vi "MasterAquisitionFile_2P_Test.vi"() -> ()   [LabVIEW 2020]
uses:
  <vilib>/userDefined/High Color/IMAQdx.ctl
  <vilib>/vision/driver/IMAQdx.llb/IMAQdx Camera Control Mode.ctl
  <vilib>/vision/driver/IMAQdx.llb/IMAQdx Acquisition Mode.ctl
  <vilib>/vision/driver/IMAQdx.llb/IMAQdx Buffer Number Mode.ctl
  <vilib>/DAQmx/write.llb/DAQmx Write (Digital 1D Wfm NChan NSamp).vi
  <vilib>/DAQmx/read.llb/DAQmx Read (Digital 1D Bool 1Chan 1Samp).vi
  <vilib>/DAQmx/read.llb/DAQmx Read (Analog 1D Wfm NChan NSamp).vi
  <vilib>/Waveform/DWDTOps.llb/DWDT Digital to Boolean Array.vi
  <vilib>/DAQmx/create/channels.llb/DAQmx Create Channel (DO-Digital Output).vi
  <vilib>/DAQmx/configure/timing.llb/DAQmx Timing (Sample Clock).vi
  <vilib>/Waveform/DWDTOps.llb/DWDT Uncompress Digital.vi
  <vilib>/DAQmx/miscellaneous.llb/DAQmx Fill In Error Info.vi
  <vilib>/DAQmx/create/channels.llb/DAQmx Create Channel (DI-Digital Input).vi
  <vilib>/DAQmx/create/channels.llb/DAQmx Create Channel (AI-Voltage-Basic).vi
  <vilib>/DAQmx/configure/trigger.llb/DAQmx Start Trigger (Digital Edge).vi
  <vilib>/DAQmx/create/channels.llb/DAQmx Create Channel (CO-Pulse Generation-Frequency).vi
  <vilib>/DAQmx/configure/timing.llb/DAQmx Timing (Implicit).vi
  <vilib>/vision/driver/NI_Vision_Acquisition_Software.lvlib
  <resource>/objmgr/imaqdx.rc
  <resource>/objmgr/daqmx.rc
panel:
  in  "Analog Input Channels":tag="Dev2/ai0:3"
  out "Auditory":bool
  out "RPad":bool
  out "LPad":bool
  in  "Sol Stim Parameters":cluster{"Fs":dbl, "Samples":dbl}
  in  "LED Stim Parameters":cluster{"Fs":dbl, "Samples":dbl}
  in  "Generate Stimuli":bool=TRUE
  in  "Sol Duty Cycle (%)":dbl=10.0
  in  "Sol Freq":dbl=10.0
  in  "Sol Dur (s)":dbl=5.0
  in  "LED Duty Cycle (%)":dbl=10.0
  in  "LED Freq":dbl=10.0
  in  "LED Dur (s)":dbl=2.0
  out "Stimulus Order":digitalwaveform[](graph)=[{"t0"=timestamp(0 s since 1904-01-01), "dt"=5e-05, "Y"={"transitions"=[], "data"=array18000000x1[18000000 elements]}}, {"t0"=timestamp(0 s since 1904-01-01), "dt"=5e-05, "Y"={"transitions"=[], "data"=array18000000x1[18000000 elements]}}, {"t0"=timestamp(0 s since 1904-01-01), "dt"=5e-05, "Y"={"transitions"=[], "data"=array18000000x1[18000000 elements]}}, {"t0"=timestamp(0 s since 1904-01-01), "dt"=5e-05, "Y"={"transitions"=[], "data"=array18000000x1[18000000 elements]}}]
  out "Solenoid Stim":digitalwaveform(graph)={"t0"=timestamp(0 s since 1904-01-01), "dt"=5e-05, "Y"={"transitions"=[], "data"=array20000x1[20000 elements]}}
  in  "Trial Offset (s)":dbl=5.0
  in  "Interstim (s)":dbl=5.0
  in  "Right Pad":dbl=1.0
  in  "Left Pad":dbl=1.0
  in  "Auditory":dbl=1.0
  in  "LED":dbl
  out "?":T1(plugin-control)
  out "MSCan Cam Fs":dbl(knob) scale=0.0..200.0
  out "MScan Cam":bool
  out "?":T1(plugin-control)
  in  "stop":bool
  out "?":T1(plugin-control)
  out "Behavior Cam Fs":dbl(knob) scale=0.0..200.0
  out "Behav Cam":bool
  out "Complete":bool
  out "Whisk Cam":bool
  out "Analog":bool
  out "MScan Trig":bool
  out "?":bool[](array[boolean])=[TRUE]
  out "Hexadecimal Data":u32=1 format="%x"
  out "Time Elapsed (Min)":cluster{dbl, dbl}(slide)={16.0, 0.028422350000000002} scale=0.0..16.0 scale format="%#_2g"
  out "Whisker Camera":bool
  out "Analog Data":bool
  out "Analog Samples":i32
  in  "Device Analog Channel Labels":string[](array[string])=["forceSensor", "AudSol", "LPadSol", "RPadSol", "", "", "", ""]
  in  "?":cluster{"Analog Fs":u16}={"Analog Fs"=20000} {"Analog Fs" format="%0.0f"}
  in  "?":cluster{"WhiskerCam Fs":u16}={"WhiskerCam Fs"=150}
  out "Notes Size":i32=7
  out "Notes Reversed":string[](array[string])=["Experimenter", "Animal ID", "Isoflurane time", "Amplifier Gain", "Session ID", "Hemisphere", "Solenoid PSI"]
  out "Notes Array":string[](array[string])=["Solenoid PSI", "Hemisphere", "Session ID", "Amplifier Gain", "Isoflurane time", "Animal ID", "Experimenter"]
  in  "Notes:":T2={"Experimenter"="Kevin\n", "Animal ID"="T201", "Isoflurane time"="1110", "Amplifier Gain"="10000", "Session ID"="Imaging Session Three", "Hemisphere"="RH", "Solenoid PSI"="10"}
  in  "Target Path":path=path "C:/Users/klt8/Documents/T201/Imaging Session 3 - 7 Apr. 2021" caption="Final Saved File Location"
  out "Dropped":u32(slide) caption="WhiskerCam" scale=0.0..150.0
  out "Current File Name":string="190611_17_21_53"
  in  "Time (min)":dbl(knob)=16.0 min=0.5 max=20.0 step=0.5 scale=0.0..20.0 scale format="%#_3g"
  in  "Temp Path":path=path "C:/Users/klt8/Documents/LabVIEW Temp Files" caption="Temporary File Path"
  out "Last Whisk Buffer":u32=251
  out "Whisker Cam Fs":dbl(knob) scale=0.0..200.0 scale format="%#1_6g"
  # "Notes"
  # "Dropped Frames"
  # "LPAD"
  # "RPAD"
  # "AUD"
  # "Analog\nFs"
  # "Whisker\nFs"
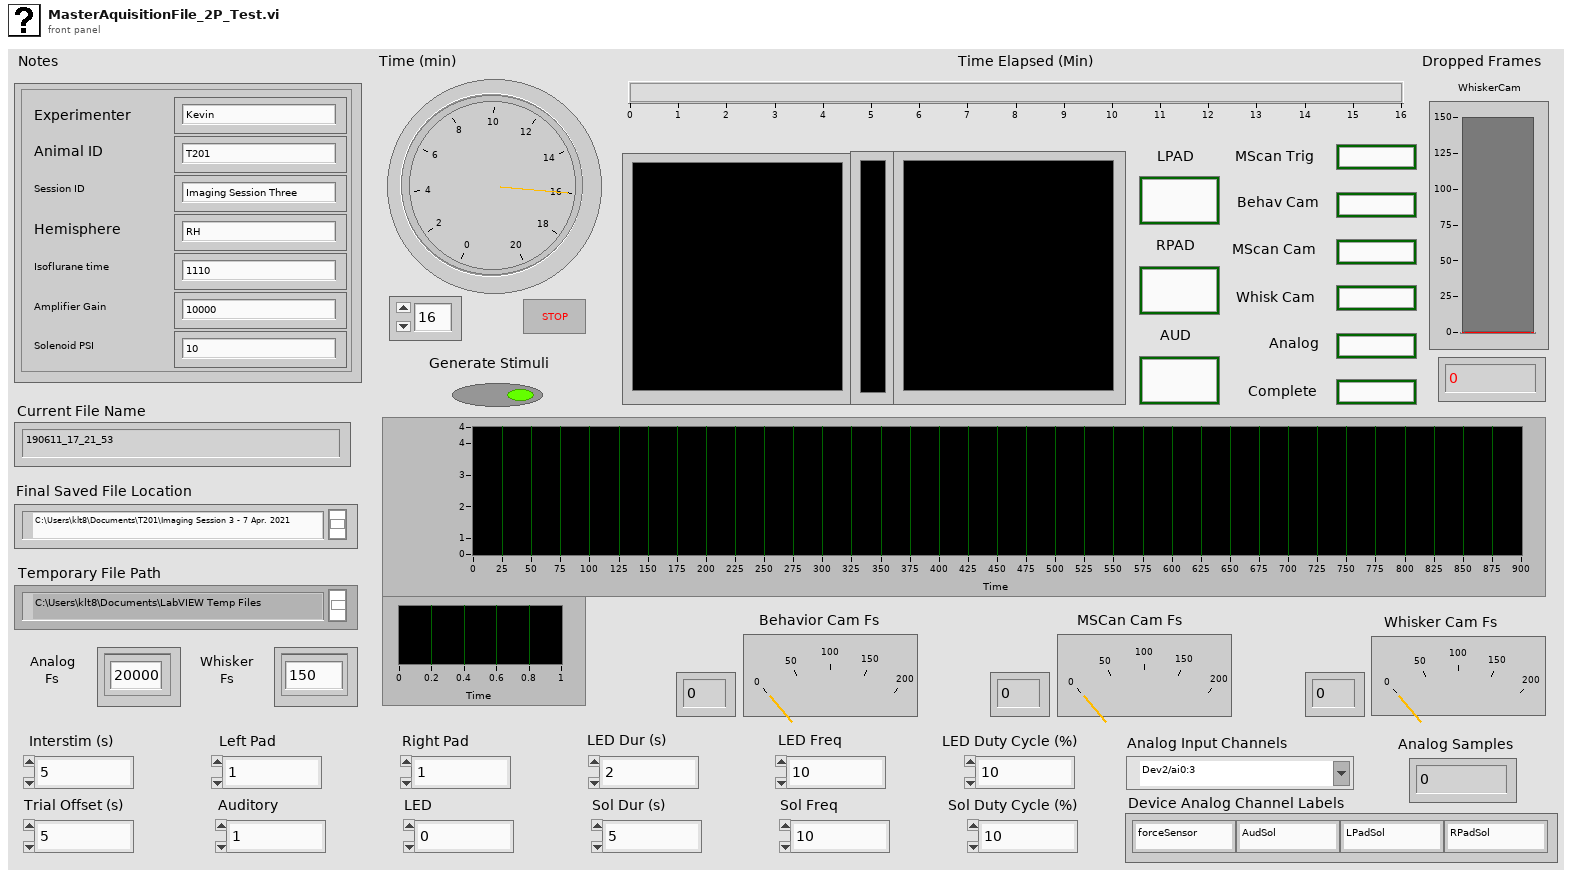
[diagram p1: front panel]
types:
  T1 = typedef "IMAQ Image.ctl" = refnum<image>
  T2 = cluster{"Experimenter":string, "Animal ID":string, "Isoflurane time":string, "Amplifier Gain":string, "Session ID":string, "Hemisphere":string, "Solenoid PSI":string}
  T3 = typedef "IMAQdx.ctl" = refnum<k21>
  T4 = typedef "NI_Vision_Acquisition_Software.lvlib/IMAQdx Camera Control Mode.ctl" = enum32{"Controller", "Listener"}
  T5 = enum16{"open", "open or create", "create or replace", "create", "open (read-only)"}
  T6 = enum16{"open", "replace", "create", "open or create", "replace or create", "replace or create with confirmation"}
  T7 = typedef "NI_Vision_Acquisition_Software.lvlib/IMAQdx Acquisition Mode.ctl" = enum32{"One Shot", "Continuous"}
  T8 = enum16{"big-endian, network order", "native, host order", "little-endian"}
  T9 = typedef "NI_Vision_Acquisition_Software.lvlib/IMAQdx Buffer Number Mode.ctl" = enum32{"Next", "Last", "Buffer Number", "Every", "Last New"}
  T10 = typedef "Image Type" = u32
  T11 = typedef "IMAQ AVI2 Refnum.ctl" = refnum<k20>
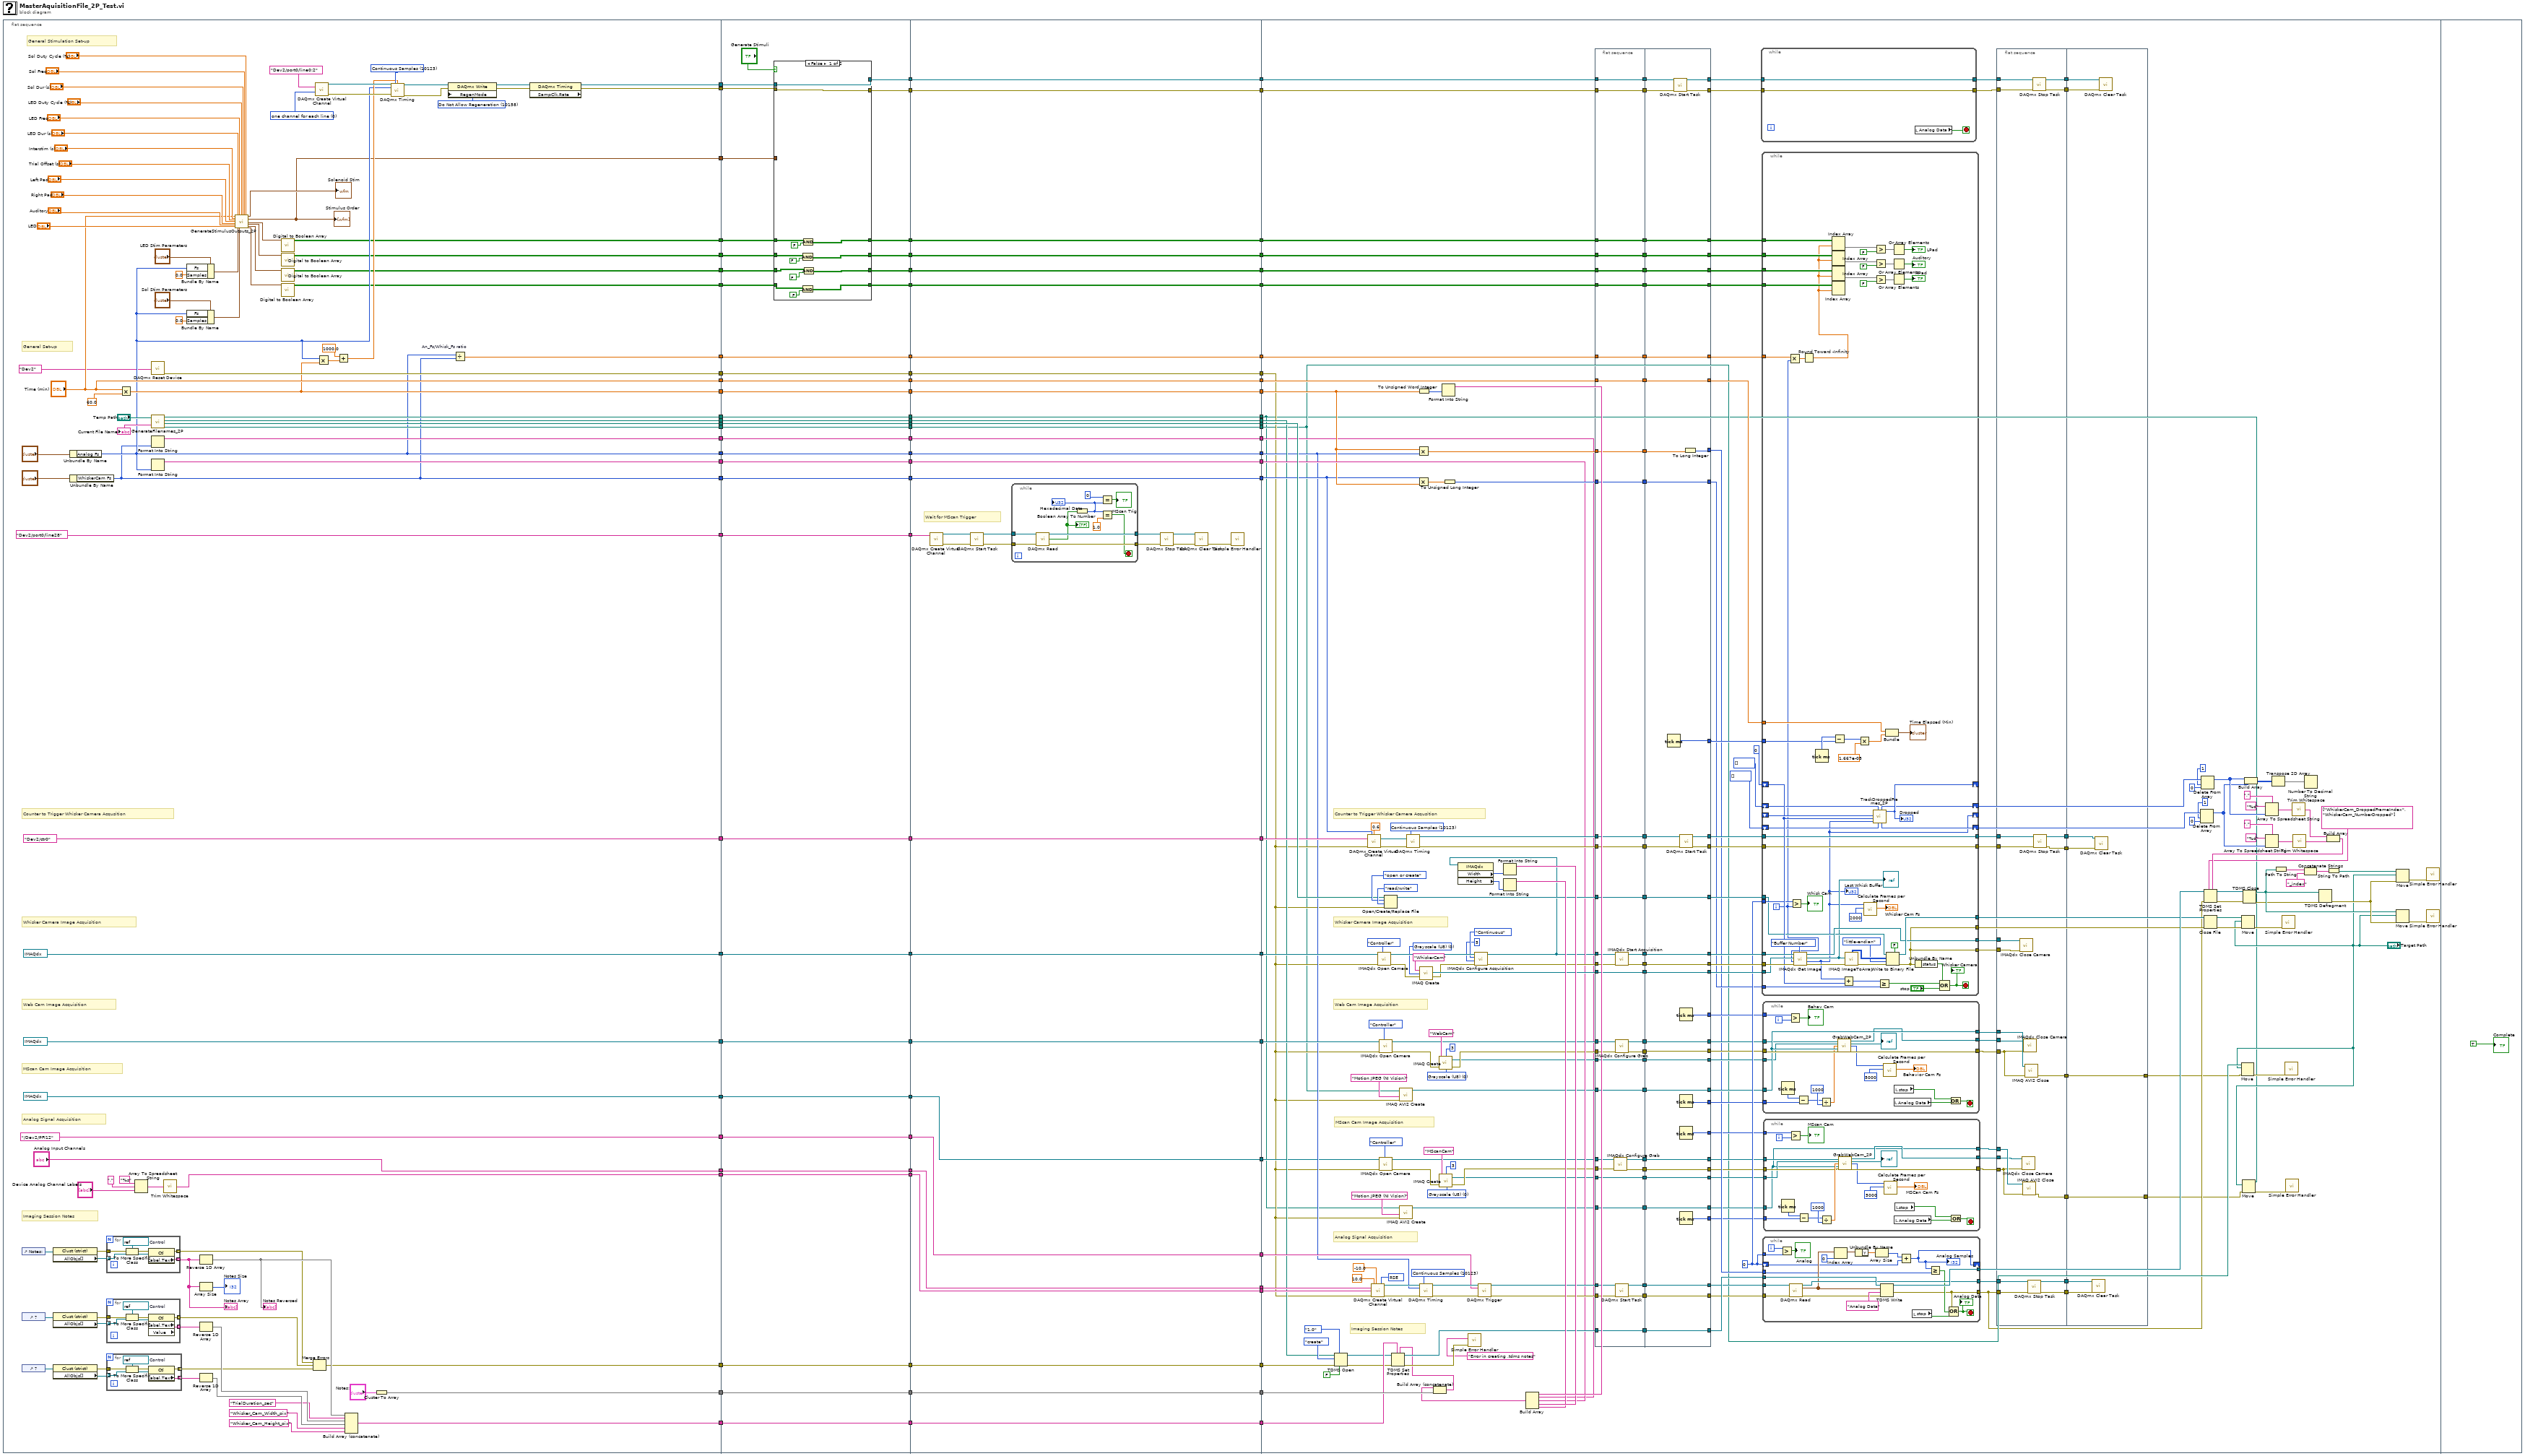
[diagram p0: block diagram]
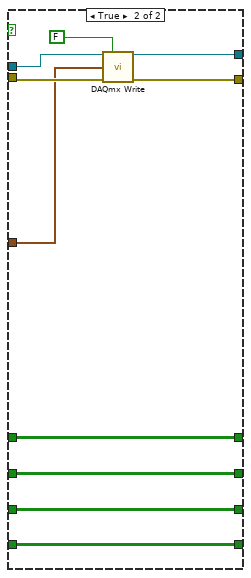
[diagram p2: hidden frame]
diagram:
  n1 = flat-sequence {
    tunnel: [tag "/Dev2/PFI12" ("Whisk Cam Trigger")] -> w59
    tunnel: [w109] -> w57
    tunnel: ["Time (min)"] -> w55
    tunnel: [w156] -> w53
    tunnel: [w155] -> w51
    tunnel: [w107] -> w49
    tunnel: [w106] -> w47
    tunnel: [w154] -> w45
    tunnel: [tag "Dev2/ctr0" ("Whisk Cam Counter")] -> w43
    tunnel: [w153] -> w41
    tunnel: ["Analog Input Channels"] -> w39
    tunnel: [T3 "cam1" ("Whisker Cam ID")] -> w37
    tunnel: [w152] -> w35
    tunnel: [w150] -> w33
    tunnel: [w151] -> w31
    tunnel: [T3 "cam2" ("WebCam ID")] -> w29
    tunnel: [tag "Dev2/port0/line28" ("MScan Trigger")] -> w27
    tunnel: [w147] -> w25
    tunnel: [w146] -> w23
    tunnel: [w145] -> w21
    tunnel: [T3 "cam7" ("WebCam ID 2")] -> w19
    tunnel: [w144] -> w17
    tunnel: [w105] -> w9
    tunnel: [w94] -> w7
    tunnel: [w93] -> w6
    tunnel: [w92] -> w5
    tunnel: [w91] -> w4
    tunnel: [w90] -> w3
    tunnel: [w89] -> w2
    tunnel: [w88] -> w1
    tunnel: w59 -> [w244]
    tunnel: [w244] -> w58
    tunnel: w57 -> [w243]
    tunnel: [w243] -> w56
    tunnel: w55 -> [w242]
    tunnel: [w242] -> w54
    tunnel: w53 -> [w241]
    tunnel: [w241] -> w52
    tunnel: w51 -> [w240]
    tunnel: [w240] -> w50
    tunnel: w49 -> [w239]
    tunnel: [w239] -> w48
    tunnel: w47 -> [w238]
    tunnel: [w238] -> w46
    tunnel: w45 -> [w237]
    tunnel: [w237] -> w44
    tunnel: w43 -> [w236]
    tunnel: [w236] -> w42
    tunnel: w41 -> [w235]
    tunnel: [w235] -> w40
    tunnel: w39 -> [w234]
    tunnel: [w234] -> w38
    tunnel: w37 -> [w233]
    tunnel: [w233] -> w36
    tunnel: w35 -> [w232]
    tunnel: [w232] -> w34
    tunnel: w33 -> [w231]
    tunnel: [w231] -> w32
    tunnel: w31 -> [w230]
    tunnel: [w230] -> w30
    tunnel: w29 -> [w229]
    tunnel: [w229] -> w28
    tunnel: w27 -> [w228]
    tunnel: [w228] -> w26
    tunnel: w25 -> [w227]
    tunnel: [w227] -> w24
    tunnel: w23 -> [w226]
    tunnel: [w226] -> w22
    tunnel: w21 -> [w225]
    tunnel: [w225] -> w20
    tunnel: w19 -> [w224]
    tunnel: [w224] -> w18
    tunnel: w17 -> [w223]
    tunnel: [w223] -> w16
    tunnel: [w214] -> w15
    tunnel: [w213] -> w14
    tunnel: [w212] -> w13
    tunnel: [w211] -> w12
    tunnel: [w210] -> w11
    tunnel: [w209] -> w10
    tunnel: w9 -> [w222]
    tunnel: [w222] -> w8
    tunnel: w7 -> [w221]
    tunnel: w6 -> [w220]
    tunnel: w5 -> [w219]
    tunnel: w4 -> [w218]
    tunnel: w3 -> [w217]
    tunnel: w2 -> [w216]
    tunnel: w1 -> [w215]
    tunnel: [w283] -> w87
    tunnel: [w295] -> w86
    tunnel: [w296] -> w85
    tunnel: [w297] -> w84
    tunnel: [w298] -> w83
    tunnel: [w285] -> w82
    tunnel: [w299] -> w81
    tunnel: [w284] -> w80
    tunnel: [w300] -> w79
    tunnel: [w301] -> w78
    tunnel: [w302] -> w77
    tunnel: [w303] -> w76
    tunnel: [w304] -> w75
    tunnel: [w305] -> w74
    tunnel: [w306] -> w73
    tunnel: w58 -> [w306]
    tunnel: w56 -> [w305]
    tunnel: w54 -> [w304]
    tunnel: w52 -> [w303]
    tunnel: w50 -> [w302]
    tunnel: w48 -> [w301]
    tunnel: w46 -> [w300]
    tunnel: w44 -> [w284]
    tunnel: w42 -> [w299]
    tunnel: w40 -> [w285]
    tunnel: w38 -> [w298]
    tunnel: w36 -> [w297]
    tunnel: w34 -> [w296]
    tunnel: w32 -> [w295]
    tunnel: w30 -> [w283]
    tunnel: [w281] -> w72
    tunnel: w28 -> [w281]
    tunnel: w26 -> [w282]
    tunnel: w24 -> [w280]
    tunnel: [w280] -> w71
    tunnel: w22 -> [w279]
    tunnel: w20 -> [w278]
    tunnel: [w279] -> w70
    tunnel: [w278] -> w69
    tunnel: w18 -> [w277]
    tunnel: [w277] -> w68
    tunnel: w16 -> [w276]
    tunnel: [w276] -> w67
    tunnel: [w275] -> w66
    tunnel: w15 -> [w275]
    tunnel: [w274] -> w65
    tunnel: w14 -> [w274]
    tunnel: [w273] -> w64
    tunnel: w13 -> [w273]
    tunnel: [w272] -> w63
    tunnel: w12 -> [w272]
    tunnel: [w271] -> w62
    tunnel: w11 -> [w271]
    tunnel: w10 -> [w270]
    tunnel: [w270] -> w61
    tunnel: [w269] -> w60
    tunnel: w8 -> [w269]
    tunnel: w87 -> [w433]
    tunnel: w86 -> [w442]
    tunnel: w85 -> [w381]
    tunnel: w84 -> [w441]
    tunnel: w83 -> [w440]
    tunnel: w82 -> [w439]
    tunnel: w81 -> [w438]
    tunnel: w80 -> [w437]
    tunnel: w79 -> [w406]
    tunnel: w78 -> [w396]
    tunnel: w77 -> [w436]
    tunnel: w76 -> [w395]
    tunnel: w75 -> [w430]
    tunnel: w74 -> [w435]
    tunnel: w73 -> [w434]
    tunnel: w72 -> [w421]
    tunnel: w71 -> [w364]
    tunnel: w70 -> [w402]
    tunnel: w69 -> [w400]
    tunnel: w68 -> [w383]
    tunnel: w67 -> [w362]
    tunnel: w66 -> [w332]
    tunnel: w65 -> [w330]
    tunnel: w64 -> [w336]
    tunnel: w63 -> [w335]
    tunnel: w62 -> [w334]
    tunnel: w61 -> [w333]
    tunnel: w60 -> [w352]
    frame #0 {
      w124 = 10158 items=["Allow Regeneration"=10097, "Do Not Allow Regeneration"=10158] ("RegenMode")
      w125 = 10123 items=["Finite Samples"=10178, "Continuous Samples"=10123, "Hardware Timed Single Point"=12522] ("sample mode")
      w128 = 0 items=["one channel for each line", "one channel for all lines"] ("line grouping")
      # "General Stimulation Set-up"
      # "MScan Cam Image Acquisition"
      # "General Set-up"
      # "Whisker Camera Image Acquisition"
      # "Imaging Session Notes"
      # "Counter to Trigger Whisker Camera Acqusition"
      # "Web Cam Image Acquisition"
      # "Analog Signal Acquisition"
      n2 = control-ref of="Notes:"() -> (w172:refnum<vi>)
      n3 = control-ref of="?"() -> (w170:refnum<vi>)
      n4 = control-ref of="?"() -> (w163:refnum<vi>)
      n5 = property class="Clust (strict)"(reference=w172) -> (error out=w171:errorcluster, "AllObjs[]"=w173:refnum<vi>[])  [unwired: 1 in, 1 out]
      n6 = property class="Clust (strict)"(reference=w170) -> (error out=w168:errorcluster, "AllObjs[]"=w169:refnum<vi>[])  [unwired: 1 in, 1 out]
      n7 = property class="Clust (strict)"(reference=w163) -> (error out=w164:errorcluster, "AllObjs[]"=w166:refnum<vi>[])  [unwired: 1 in, 1 out]
      n8 = Unbundle By Name("?") -> ("Analog Fs"=w107:u16)
      n9 = Unbundle By Name("?") -> ("WhiskerCam Fs"=w106:u16)
      n10 = for {
        tunnel: [w191] -> w178 mode=indexing
        tunnel: w173 -> [w190] mode=indexing
        tunnel: w171 -> [w189]
        tunnel: [w187] -> w177 mode=indexing
        w192 = refnum<vi> refnum  # Control
        n11 = To More Specific Class(target class=w192, reference=w190, error in=w189) -> (specific class reference=w193:refnum<vi>, error out=w188:errorcluster)
        n12 = property class="Ctl"(reference=w193, error in=w188) -> (error out=w187:errorcluster, "Label.Text"=w191:string)  [unwired: 1 out]
      }
      "Notes Array" <- w178
      n13 = for {
        tunnel: [w198] -> w167 mode=indexing
        tunnel: w169 -> [w197] mode=indexing
        tunnel: w168 -> [w196]
        tunnel: [w194] -> w176 mode=indexing
        w199 = refnum<vi> refnum  # Control
        n14 = To More Specific Class(target class=w199, reference=w197, error in=w196) -> (specific class reference=w200:refnum<vi>, error out=w195:errorcluster)
        n15 = property class="Ctl" props=["Label", "Text", "Value"](reference=w200, error in=w195) -> (error out=w194:errorcluster, "Label.Text"=w198:string)  [unwired: 2 out]
      }
      n16 = for {
        tunnel: [w205] -> w165 mode=indexing
        tunnel: w166 -> [w204] mode=indexing
        tunnel: w164 -> [w203]
        tunnel: [w201] -> w175 mode=indexing
        w206 = refnum<vi> refnum  # Control
        n17 = To More Specific Class(target class=w206, reference=w204, error in=w203) -> (specific class reference=w207:refnum<vi>, error out=w202:errorcluster)
        n18 = property class="Ctl"(reference=w207, error in=w202) -> (error out=w201:errorcluster, "Label.Text"=w205:string)  [unwired: 1 out]
      }
      n19 = Multiply(x="Time (min)", y=60.0) -> (x*y=w109:dbl)
      n20 = Array To Spreadsheet String(delimiter (Tab)=",", array="Device Analog Channel Labels", 3:"%s" ("format string")) -> (spreadsheet string=w180:string)
      n21 = call <vilib>:"DAQmx Reset Device.vi"("device in"=tag "Dev2" ("NI Board")) -> ("error out"=w152:errorcluster)  [unwired: 14 in]
      n22 = call "GenerateFilenames_2P.vi"("path"="Temp Path") -> ("WebCam Path"=w147:path, "Basler Path"=w150:path, "TDMS Path"=w145:path, "MScan Path"=w144:path, "Analog file name"=→"Current File Name":string)  [unwired: 2 in]
      n23 = Format Into String(w106) -> (resulting string=w156:string)  [unwired: 3 in, 1 out]
      n24 = Format Into String(w107) -> (resulting string=w155:string)  [unwired: 3 in, 1 out]
      n25 = call <vilib>:"Trim Whitespace.vi"("string"=w180) -> ("trimmed string"=w153:string)  [unwired: 1 in]
      n26 = Bundle By Name(cluster="LED Stim Parameters", "Fs"=w107, "Samples"=0.0) -> (w114:cluster{"Fs":dbl, "Samples":dbl})
      n27 = Bundle By Name(cluster="Sol Stim Parameters", "Fs"=w107, "Samples"=0.0) -> (w113:cluster{"Fs":dbl, "Samples":dbl})
      n28 = Reverse 1D Array(array=w178) -> (reversed array=w179:string[])
      "Notes Reversed" <- w179
      n29 = Array Size(array=w178) -> (size(s)=→"Notes Size":i32)
      n30 = Reverse 1D Array(array=w167) -> (reversed array=w185:string[])
      n31 = Reverse 1D Array(array=w165) -> (reversed array=w186:string[])
      n32 = call "GenerateStimulusOutputs_2P.vi"("Trial duration (min)"="Time (min)", "Rest duration(s)"="Interstim (s)", "trial offset (s)"="Trial Offset (s)", "Left Pad"="Left Pad", "Right Pad"="Right Pad", "Auditory"="Auditory", "LED"="LED", "LED Stim Duration (s)"="LED Dur (s)", "LED Stim Parameters"=w114, "LED Frequency"="LED Freq", "Sol Stim Parameters"=w113, "LED duty cycle (%)"="LED Duty Cycle (%)", "Sol Stim Duration (s)"="Sol Dur (s)", "Sol Frequency"="Sol Freq", "Sol Duty Cycle (%)"="Sol Duty Cycle (%)") -> ("Solenoid Stim Waveforms"=→"Solenoid Stim":digitalwaveform, "Stimulus Digital Outputs"=w90:digitalwaveform[], "Left Pad Out"=w103:digitalwaveform, "Auditory Out"=w130:digitalwaveform, "Right Pad Out"=w129:digitalwaveform, "LED Out"=w108:digitalwaveform)  [unwired: 7 in]
      "Stimulus Order" <- w90
      n33 = call-poly <vilib>:"Digital to Boolean Array.vi"("digital waveform"=w103) -> ("boolean array"=w89:bool[][])  [unwired: 9 in, 1 out]
      n34 = call-poly <vilib>:"Digital to Boolean Array.vi"("digital waveform"=w130) -> ("boolean array"=w92:bool[][])  [unwired: 9 in, 1 out]
      n35 = call-poly <vilib>:"Digital to Boolean Array.vi"("digital waveform"=w129) -> ("boolean array"=w91:bool[][])  [unwired: 9 in, 1 out]
      n36 = call-poly <vilib>:"Digital to Boolean Array.vi"("digital waveform"=w108) -> ("boolean array"=w88:bool[][])  [unwired: 9 in, 1 out]
      n37 = Merge Errors(w177, w176, w175) -> (w146:errorcluster)
      n38 = call-poly <vilib>:"DAQmx Create Virtual Channel.vi"("lines"=tag "Dev2/port0/line0:2", "line grouping"=w128) -> ("task out"=w127:refnum<k21>, "error out"=w126:errorcluster)  [unwired: 12 in]
      n39 = Multiply(x=w107, y=w109) -> (x*y=w112:dbl)
      n40 = Add(x=1000.0, y=w112) -> (x+y=w110:dbl)
      n41 = Build Array (concatenate)(w179, "TrialDuration_sec", w185, w186, "Whisker_Cam_Width_pix", "Whisker_Cam_Height_pix") -> (w151:string[])
      n42 = Cluster To Array(cluster="Notes:") -> (array=w154:string[])
      n43 = call-poly <vilib>:"DAQmx Timing.vi"("task/channels in"=w127, "sample mode"=w125, "samples per channel"=w110, "rate"=w107, "error in"=w126) -> ("task out"=w121:refnum<k21>, "error out"=w120:errorcluster)  [unwired: 9 in]
      n44 = property class="DAQmx Write"(reference=w121, error in=w120, "RegenMode"=w124) -> (reference out=w122:refnum<k21>, error out=w123:errorcluster)
      n45 = Divide "An_Fs/Whisk_Fs ratio"(x=w107, y=w106) -> (x/y=w105:dbl)
      n46 = property class="DAQmx Timing" props=["SampClk.Rate"](reference=w122, error in=w123) -> (reference out=w94:refnum<k21>, error out=w93:errorcluster)  [unwired: 1 out]
    }
    frame #1 {
      n47 = case shown="False" "Generate Stimuli" {
        tunnel: w221 -> [w258 w268]
        tunnel: w220 -> [w257 w267]
        tunnel: [w258 w266] -> w214
        tunnel: [w257 w265] -> w213
        tunnel: w219 -> [w253 w264]
        tunnel: w218 -> [w254 w263]
        tunnel: [w247 w261] -> w212
        tunnel: [w256 w264] -> w211
        tunnel: [w255 w263] -> w210
        tunnel: [w246 w260] -> w209
        tunnel: w217 -> [_ w262]
        tunnel: w216 -> [w248 w261]
        tunnel: w215 -> [w245 w260]
        frame False {
          n48 = Compound Arithmetic op=AND(w253, FALSE) -> (w256:bool[][])
          n49 = Compound Arithmetic op=AND(w245, FALSE) -> (w246:bool[][])
          n50 = Compound Arithmetic op=AND(w248, FALSE) -> (w247:bool[][])
          n51 = Compound Arithmetic op=AND(w254, FALSE) -> (w255:bool[][])
        }
        frame True {
          n52 = call-poly <vilib>:"DAQmx Write.vi"("task/channels in"=w268, "auto start"=FALSE, "data"=w262, "error in"=w267) -> ("task out"=w266:refnum<k21>, "error out"=w265:errorcluster)  [unwired: 9 in, 1 out]
        }
      }
    }
    frame #2 {
      # "Wait for MScan Trigger"
      n53 = call-poly <vilib>:"DAQmx Create Virtual Channel.vi"("lines"=w282) -> ("task out"=w290:refnum<k21>, "error out"=w291:errorcluster)  [unwired: 13 in]
      n54 = call <vilib>:"DAQmx Start Task.vi"("task/channels in"=w290, "error in"=w291) -> ("task out"=w294:refnum<k21>, "error out"=w293:errorcluster)  [unwired: 12 in]
      n55 = while {
        tunnel: w294 -> [w316]
        tunnel: w293 -> [w315]
        tunnel: [w313] -> w288
        tunnel: [w314] -> w289
        stop <- w308 stop-if-true
        n56 = call-poly <vilib>:"DAQmx Read.vi"("task/channels in"=w316, "error in"=w315) -> ("task out"=w314:refnum<k21>, "data"=w312:bool[], "error out"=w313:errorcluster)  [unwired: 11 in]
        "?" <- w312
        n57 = Boolean Array To Number(Boolean array=w312) -> (number=w307:u32)
        "Hexadecimal Data" <- w307
        n58 = Equal?(x=w307, y=u32 0) -> (x = y?=→"MScan Trig":bool)
        n59 = Equal?(x=w307, y=1.0) -> (x = y?=w308:bool)
      }
      n60 = call <vilib>:"DAQmx Stop Task.vi"("task/channels in"=w289, "error in"=w288) -> ("task out"=w287:refnum<k21>, "error out"=w286:errorcluster)  [unwired: 12 in]
      n61 = call <vilib>:"DAQmx Clear Task.vi"("task in"=w287, "error in"=w286) -> ("error out"=w292:errorcluster)  [unwired: 13 in]
      n62 = call <vilib>:"Simple Error Handler.vi"("error in (no error)"=w292) -> ()  [unwired: 4 in, 5 out]
    }
    frame #3 {
      w386 = T10 0 items=["Grayscale (U8)", "Grayscale (I16)", "Grayscale (SGL)", "Complex (CSG)", "RGB (U32)", "HSL (U32)", "RGB (U64)", "Grayscale (U16)"] ("Image Type")
      w425 = T10 0 items=["Grayscale (U8)", "Grayscale (I16)", "Grayscale (SGL)", "Complex (CSG)", "RGB (U32)", "HSL (U32)", "RGB (U64)", "Grayscale (U16)"] ("Image Type")
      w413 = u32 0 ("y")
      w451 = 10123 items=["Finite Samples"=10178, "Continuous Samples"=10123, "Hardware Timed Single Point"=12522] ("sample mode")
      w450 = 10083 items=["default"=-1, "RSE"=10083, "NRSE"=10078, "Differential"=10106, "Pseudodifferential"=12529] ("input terminal configuration")
      w452 = 10123 items=["Finite Samples"=10178, "Continuous Samples"=10123, "Hardware Timed Single Point"=12522] ("sample mode")
      w448 = T10 0 items=["Grayscale (U8)", "Grayscale (I16)", "Grayscale (SGL)", "Complex (CSG)", "RGB (U32)", "HSL (U32)", "RGB (U64)", "Grayscale (U16)"] ("Image Type")
      # "MScan Cam Image Acquisition"
      # "Whisker Camera Image Acquisition"
      # "Imaging Session Notes"
      # "Counter to Trigger Whisker Camera Acqusition"
      # "Web Cam Image Acquisition"
      # "Analog Signal Acquisition"
      n63 = TDMS Open(6:FALSE ("disable buffering? (T)"), 7:enum16{"1.0", "2.0"}."1.0" ("file format version (2.0)"), 8:w402, 10:T5."create" ("operation (0:open)"), 11:w400) -> (0:w399:errorcluster, 3:w398:refnum<k34>)  [unwired: 2 in]
      n64 = call-poly <vilib>:"DAQmx Create Virtual Channel.vi"("frequency"=w406, "duty cycle"=0.6, "counter"=w438, "error in"=w381) -> ("task out"=w475:refnum<k21>, "error out"=w476:errorcluster)  [unwired: 10 in]
      n65 = call-poly <vilib>:"DAQmx Create Virtual Channel.vi"("maximum value"=10.0, "minimum value"=-10.0, "input terminal configuration"=w450, "physical channels"=w440, "name to assign"=w439, "error in"=w381) -> ("task out"=w484:refnum<k21>, "error out"=w485:errorcluster)  [unwired: 8 in]
      n66 = call <vilib>:"IMAQdx Open Camera.vi"("Camera Control Mode"=IMAQdx_Camera_Control_Mode."Controller", "error in"=w381, "Session In"=w441) -> ("error out"=w473:errorcluster, "Session Out"=w472:T3)  [unwired: 7 in]
      n67 = call <vilib>:"IMAQdx Open Camera.vi"("Camera Control Mode"=IMAQdx_Camera_Control_Mode."Controller", "error in"=w381, "Session In"=w421) -> ("error out"=w422:errorcluster, "Session Out"=w420:T3)  [unwired: 7 in]
      n68 = call <vilib>:"IMAQdx Open Camera.vi"("Camera Control Mode"=IMAQdx_Camera_Control_Mode."Controller", "error in"=w381, "Session In"=w383) -> ("error out"=w384:errorcluster, "Session Out"=w378:T3)  [unwired: 7 in]
      n69 = Open/Create/Replace File(file path (use dialog)=w442, error in=w381, operation (0:open)=T6."open or create", access (0:read/write)=enum16{"read/write", "read-only", "write-only"}."read/write") -> (refnum out=w483:refnum<file>)  [unwired: 2 in, 2 out]
      n70 = call "IMAQ AVI2 Create"("error in (no error)"=w381, "Codec"="Motion JPEG (NI Vision)", "AVI Path"=w364) -> ("AVI Refnum"=w408:T11)  [unwired: 7 in, 1 out]
      n71 = call "IMAQ AVI2 Create"("error in (no error)"=w381, "Codec"="Motion JPEG (NI Vision)", "AVI Path"=w362) -> ("AVI Refnum"=w374:T11)  [unwired: 7 in, 1 out]
      n72 = call-poly <vilib>:"DAQmx Timing.vi"("task/channels in"=w475, "sample mode"=w452, "error in"=w476) -> ("task out"=w493:refnum<k21>, "error out"=w494:errorcluster)  [unwired: 11 in]
      n73 = Multiply(x=w435, y=w396) -> (x*y=w520:dbl)
      n74 = Multiply(x=w406, y=w435) -> (x*y=w521:dbl)
      n75 = To Unsigned Word Integer(number=w435) -> (unsigned 16bit integer=w508:u16)
      n76 = call "IMAQ Create"("Image Name"="WhiskerCam", "Image Type"=w448, "error in (no error)"=w473) -> ("New Image"=w511:T1, "error out"=w474:errorcluster)  [unwired: 2 in]
      n77 = call-poly <vilib>:"DAQmx Timing.vi"("task/channels in"=w484, "sample mode"=w451, "rate"=w396, "error in"=w485) -> ("task out"=w486:refnum<k21>, "error out"=w487:errorcluster)  [unwired: 10 in]
      n78 = call "IMAQ Create"("Border Size"=3, "Image Name"="WebCam", "Image Type"=w425, "error in (no error)"=w422) -> ("New Image"=w418:T1, "error out"=w419:errorcluster)  [unwired: 1 in]
      n79 = call "IMAQ Create"("Border Size"=3, "Image Name"="MScanCam", "Image Type"=w386, "error in (no error)"=w384) -> ("New Image"=w368:T1, "error out"=w379:errorcluster)  [unwired: 1 in]
      n80 = Format Into String(w508) -> (resulting string=w529:string)  [unwired: 3 in, 1 out]
      n81 = To Unsigned Long Integer(number=w521) -> (unsigned 32bit integer=w522:u32)
      n82 = call <vilib>:"IMAQdx Configure Acquisition.vi"("error in"=w474, "Number of Buffers"=u32 5, "Continuous?"=IMAQdx_Acquisition_Mode."Continuous", "Session In"=w472) -> ("error out"=w478:errorcluster, "Session Out"=w397:T3)  [unwired: 6 in]
      n83 = property class="IMAQdx"(reference=w397) -> ("Width"=w509:u32, "Height"=w510:u32)  [unwired: 1 in, 2 out]
      n84 = call-poly <vilib>:"DAQmx Trigger.vi"("task/channels in"=w486, "source"=w434, "error in"=w487) -> ("task out"=w488:refnum<k21>, "error out"=w489:errorcluster)  [unwired: 11 in]
      n85 = Format Into String(w509) -> (resulting string=w528:string)  [unwired: 3 in, 1 out]
      n86 = Format Into String(w510) -> (resulting string=w527:string)  [unwired: 3 in, 1 out]
      n87 = Build Array(w529, w395, w436, w528, w527) -> (w393:string[])
      n88 = Build Array (concatenate)(w437, w393) -> (w443:string[])
      n89 = TDMS Set Properties(5:w443, 7:w433, 8:w399, 11:w398) -> (0:w507:errorcluster, 3:w506:refnum<k34>)  [unwired: 2 in, 2 out]
      n90 = call <vilib>:"Simple Error Handler.vi"("error source (\" \")"="Error in creating .tdms notes" ("error source (\" \")"), "error in (no error)"=w507) -> ()  [unwired: 3 in, 5 out]
      n91 = flat-sequence {
        tunnel: w397 -> [w672]
        tunnel: w478 -> [w671]
        tunnel: [w670] -> w540
        tunnel: [w669] -> w539
        tunnel: [w668] -> w538
        tunnel: w511 -> [w668]
        tunnel: [w667] -> w537
        tunnel: w483 -> [w667]
        tunnel: w488 -> [w666]
        tunnel: w489 -> [w665]
        tunnel: [w664] -> w536
        tunnel: [w663] -> w535
        tunnel: [w662] -> w534
        tunnel: w506 -> [w662]
        tunnel: w493 -> [w661]
        tunnel: [w661] -> w533
        tunnel: w494 -> [w660]
        tunnel: [w660] -> w532
        tunnel: w520 -> [w659]
        tunnel: [w659] -> w531
        tunnel: w522 -> [w658]
        tunnel: [w658] -> w530
        tunnel: w430 -> [w657]
        tunnel: [w657] -> w429
        tunnel: w420 -> [w656]
        tunnel: w419 -> [w655]
        tunnel: w418 -> [w654]
        tunnel: [w654] -> w417
        tunnel: [w653] -> w416
        tunnel: [w652] -> w415
        tunnel: [w651] -> w409
        tunnel: w408 -> [w651]
        tunnel: w379 -> [w647]
        tunnel: w378 -> [w650]
        tunnel: [w649] -> w377
        tunnel: [w648] -> w376
        tunnel: [w646] -> w375
        tunnel: w374 -> [w646]
        tunnel: [w645] -> w369
        tunnel: w368 -> [w645]
        tunnel: [w644] -> w361
        tunnel: w336 -> [w644]
        tunnel: [w643] -> w360
        tunnel: w335 -> [w643]
        tunnel: [w642] -> w359
        tunnel: w334 -> [w642]
        tunnel: [w641] -> w358
        tunnel: w333 -> [w641]
        tunnel: [w640] -> w353
        tunnel: w352 -> [w640]
        tunnel: w332 -> [w638]
        tunnel: [w639] -> w331
        tunnel: w330 -> [w639]
        tunnel: [w638] -> w329
        tunnel: [w702] -> w431
        tunnel: [w701] -> w432
        tunnel: [w709] -> w479
        tunnel: w540 -> [w709]
        tunnel: [w708] -> w480
        tunnel: w539 -> [w708]
        tunnel: [w707] -> w481
        tunnel: w538 -> [w707]
        tunnel: [w706] -> w482
        tunnel: w537 -> [w706]
        tunnel: [w705] -> w491
        tunnel: w536 -> [w705]
        tunnel: [w704] -> w490
        tunnel: w535 -> [w704]
        tunnel: [w703] -> w492
        tunnel: w534 -> [w703]
        tunnel: w533 -> [w698]
        tunnel: w532 -> [w700]
        tunnel: w531 -> [w689]
        tunnel: w530 -> [w699]
        tunnel: [w699] -> w392
        tunnel: [w697] -> w471
        tunnel: w429 -> [w696]
        tunnel: [w696] -> w428
        tunnel: [w695] -> w412
        tunnel: w417 -> [w695]
        tunnel: [w694] -> w410
        tunnel: w416 -> [w694]
        tunnel: [w693] -> w411
        tunnel: w415 -> [w693]
        tunnel: [w692] -> w405
        tunnel: w409 -> [w691]
        tunnel: [w691] -> w407
        tunnel: [w690] -> w404
        tunnel: [w688] -> w391
        tunnel: [w687] -> w371
        tunnel: w377 -> [w687]
        tunnel: [w686] -> w370
        tunnel: w376 -> [w686]
        tunnel: [w685] -> w365
        tunnel: w375 -> [w685]
        tunnel: [w684] -> w373
        tunnel: [w683] -> w372
        tunnel: w369 -> [w682]
        tunnel: [w682] -> w367
        tunnel: w361 -> [w681]
        tunnel: [w681] -> w357
        tunnel: [w680] -> w356
        tunnel: w360 -> [w680]
        tunnel: w359 -> [w679]
        tunnel: [w679] -> w355
        tunnel: w358 -> [w678]
        tunnel: [w678] -> w354
        tunnel: [w677] -> w351
        tunnel: w353 -> [w677]
        tunnel: [w676] -> w350
        tunnel: [w675] -> w349
        tunnel: w331 -> [w674]
        tunnel: w329 -> [w673]
        frame #0 {
          n92 = call <vilib>:"IMAQdx Configure Grab.vi"("error in"=w647, "Session In"=w650) -> ("error out"=w648:errorcluster, "Session Out"=w649:T3)  [unwired: 8 in]
          n93 = call <vilib>:"IMAQdx Start Acquisition.vi"("error in"=w671, "Session In"=w672) -> ("error out"=w669:errorcluster, "Session Out"=w670:T3)  [unwired: 8 in]
          n94 = call <vilib>:"IMAQdx Configure Grab.vi"("error in"=w655, "Session In"=w656) -> ("error out"=w652:errorcluster, "Session Out"=w653:T3)  [unwired: 8 in]
          n95 = call <vilib>:"DAQmx Start Task.vi"("task/channels in"=w666, "error in"=w665) -> ("task out"=w664:refnum<k21>, "error out"=w663:errorcluster)  [unwired: 12 in]
        }
        frame #1 {
          n96 = Tick Count (ms)() -> (millisecond timer value=w697:u32)
          n97 = call <vilib>:"DAQmx Start Task.vi"("task/channels in"=w673, "error in"=w674) -> ("task out"=w676:refnum<k21>, "error out"=w675:errorcluster)  [unwired: 12 in]
          n98 = Tick Count (ms)() -> (millisecond timer value=w692:u32)
          n99 = Tick Count (ms)() -> (millisecond timer value=w690:u32)
          n100 = Tick Count (ms)() -> (millisecond timer value=w683:u32)
          n101 = Tick Count (ms)() -> (millisecond timer value=w684:u32)
          n102 = call <vilib>:"DAQmx Start Task.vi"("task/channels in"=w698, "error in"=w700) -> ("task out"=w702:refnum<k21>, "error out"=w701:errorcluster)  [unwired: 12 in]
          n103 = To Long Integer(number=w689) -> (32bit integer=w688:i32)
        }
      }
      n104 = while {
        tunnel: w350 -> [w573]
        tunnel: [w571] -> w345
        tunnel: w349 -> [w571]
        tunnel: [w573] -> w346
        stop <- w572 stop-if-true
        n105 = local read "Analog Data"() -> (w572:bool)
      }
      n106 = while {
        tunnel: [w755] -> w327
        tunnel: [w739] -> w505
        tunnel: [w763] -> w477
        tunnel: w479 -> [w762]
        tunnel: w480 -> [w761]
        tunnel: w481 -> [w760]
        tunnel: w482 -> [w733]
        shift-right: [w713] -> _
        shift-left: _ -> [w759]
        shift-right: [w758] -> _
        shift-left: u32 0 ("New Lost") -> [w754]
        shift-right: [w757] -> w519
        shift-left: u32[] [] ("NewBuffNum") -> [w712]
        shift-right: [w756] -> w495
        shift-left: u32[] [] ("NewNumLost") -> [w748]
        tunnel: w392 -> [w752]
        tunnel: w471 -> [w743]
        tunnel: w428 -> [w741]
        tunnel: [w739] -> w328
        tunnel: w413 -> [w738]
        tunnel: w432 -> [w736]
        tunnel: w431 -> [w735]
        tunnel: [w736] -> w343
        tunnel: [w735] -> w344
        tunnel: w357 -> [w719]
        tunnel: w356 -> [w718]
        tunnel: w355 -> [w717]
        tunnel: w354 -> [w716]
        tunnel: w351 -> [w714]
        i -> [w710]
        stop <- w749 stop-if-true
        n107 = Multiply(x=w714, y=w710) -> (x*y=w715:dbl)
        n108 = Greater?(x=w710, y=w738) -> (0:→"Whisk Cam":bool)
        n109 = call <vilib>:"IMAQdx Get Image.vi"("Buffer Number Mode (Next)"=IMAQdx_Buffer_Number_Mode."Buffer Number", "error in"=w761, "Buffer Number In"=w710, "Image In"=w760, "Session In"=w762) -> ("error out"=w769:errorcluster, "Buffer Number Out"=w713:u32, "Image Out"=w732:T1, "Session Out"=w755:T3)  [unwired: 3 in]
        "Last Whisk Buffer" <- w713
        "?" <- w732
        n110 = Round Toward -Infinity(1:w715) -> (0:w711:dbl)
        n111 = Tick Count (ms)() -> (millisecond timer value=w744:u32)
        n112 = Index Array(array=w719, index (row)=w711) -> (element=w725:bool[])  [unwired: 1 in]
        n113 = Index Array(array=w718, index (row)=w711) -> (element=w723:bool[])  [unwired: 1 in]
        n114 = Index Array(array=w717, index (row)=w711) -> (element=w721:bool[])  [unwired: 1 in]
        n115 = Index Array(array=w716, index (row)=w711) -> ()  [unwired: 1 in, 1 out]
        n116 = Subtract(x=w744, y=w743) -> (x-y=w747:u32)
        n117 = Add(x=w713, y=w754) -> (x+y=w753:u32)
        n118 = call "IMAQ ImageToArray"("error in (no error)"=w769, "Image"=w732) -> ("error out"=w768:errorcluster, "Image Pixels (U8)"=w767:u8[][])  [unwired: 2 in, 3 out]
        n119 = Multiply(x=w747, y=1.667e-05) -> (x*y=w746:dbl)
        n120 = call <vilib>:"Calculate Frames per Second.vi"("Update Interval (ms)"=u32 2000, "Buffer Number"=w713) -> ("Processed Frames/s"=→"Whisker Cam Fs":dbl)  [unwired: 7 in, 2 out]
        n121 = call "TrackDroppedFrames_2P.vi"("NumLost"=w748, "BuffNum"=w712, "Curr Buffer"=w713, "Prev Lost"=w754, "Prev Buffer"=w759) -> ("New Lost"=w758:u32, "NewNumLost"=w756:u32[], "NewBuffNum"=w757:u32[])  [unwired: 4 in]
        "Dropped" <- w758
        n122 = Greater?(x=w725, y=FALSE ("Boolean")) -> (0:w724:bool[])
        n123 = Greater?(x=w723, y=FALSE ("Boolean")) -> (0:w722:bool[])
        n124 = Greater?(x=w721, y=FALSE ("Boolean")) -> (0:w720:bool[])
        n125 = Greater Or Equal?(x=w753, y=w752) -> (x >= y?=w750:bool)
        n126 = Bundle("Time (min)"=w741, w746) -> (→"Time Elapsed (Min)":cluster{"Time (min)":dbl, dbl})  [unwired: 1 in]
        n127 = Write to Binary File(file (use dialog)=w733, data=w767, error in=w768, 5:FALSE ("prepend array or string size? (T)"), 9:T8."little-endian" ("byte order (0:big-endian, network order)")) -> (refnum out=w763:refnum<file>, error out=w739:errorcluster)  [unwired: 1 in, 1 out]
        n128 = Or Array Elements(Boolean array=w724) -> (logical OR=→"LPad":bool)
        n129 = Or Array Elements(Boolean array=w722) -> (logical OR=→"Auditory":bool)
        n130 = Or Array Elements(Boolean array=w720) -> (logical OR=→"RPad":bool)
        n131 = Unbundle By Name(w739) -> ("status"=w751:bool)
        n132 = Compound Arithmetic op=OR(w751, w750, "stop") -> (w749:bool)
        "Whisker Camera" <- w749
      }
      n133 = while {
        tunnel: w490 -> [w637]
        tunnel: w491 -> [w636]
        tunnel: w492 -> [w635]
        tunnel: [w634] -> w512
        tunnel: [w622] -> w337
        tunnel: [w633] -> w338
        shift-right: [w626] -> _
        shift-left: w413 -> [w627]
        tunnel: w413 -> [w618]
        tunnel: w391 -> [w616]
        i -> [w619]
        stop <- w623 stop-if-true
        n134 = Greater?(x=w619, y=w618) -> (0:→"Analog":bool)
        n135 = call-poly <vilib>:"DAQmx Read.vi"("task/channels in"=w636, "error in"=w637) -> ("task out"=w633:refnum<k21>, "data"=w631:waveform(dbl)[], "error out"=w625:errorcluster)  [unwired: 11 in]
        n136 = Index Array(array=w631, index=0) -> (element=w629:waveform(dbl))
        n137 = Unbundle By Name(w629) -> ("Y"=w628:dbl[])
        n138 = Array Size(array=w628) -> (size(s)=w621:i32)
        n139 = TDMS Write(0:w635, 5:"Analog Data" ("group name in (Untitled)"), 9:w631, 11:w625) -> (4:w634:refnum<k34>, 15:w622:errorcluster)  [unwired: 2 in, 2 out]
        n140 = Add(x=w621, y=w627) -> (x+y=w626:u32)
        "Analog Samples" <- w626
        n141 = local read "stop"() -> (w617:bool)
        n142 = Greater Or Equal?(x=w626, y=w616) -> (x >= y?=w624:bool)
        n143 = Compound Arithmetic op=OR(w617, w622, w624) -> (w623:bool)
        "Analog Data" <- w623
      }
      n144 = while {
        tunnel: w412 -> [w602]
        tunnel: w410 -> [w601]
        tunnel: w411 -> [w605]
        tunnel: w407 -> [w604]
        tunnel: [w595] -> w324
        tunnel: [w606] -> w326
        tunnel: [w604] -> w325
        tunnel: w405 -> [w608]
        tunnel: w404 -> [w607]
        i -> [w609]
        stop <- w597 stop-if-true
        n145 = Tick Count (ms)() -> (millisecond timer value=w613:u32)
        n146 = Greater?(x=w608, y=w609) -> (0:→"Behav Cam":bool)
        n147 = Subtract(x=w613, y=w607) -> (x-y=w614:u32)
        n148 = Divide(x=w614, y=u32 1000) -> (x/y=w603:dbl)
        n149 = call "GrabWebCam_2P.vi"("Session In"=w601, "Image In"=w602, "Trial Time"=w603, "AVI Refnum"=w604, "error in"=w605) -> ("Session Out"=w595:T3, "WebCam Img Out"=→"?":T1, "Buffer Number Out"=w599:u32, "error out"=w606:errorcluster)  [unwired: 7 in]
        n150 = call <vilib>:"Calculate Frames per Second.vi"("Update Interval (ms)"=u32 5000, "Buffer Number"=w599) -> ("Processed Frames/s"=→"Behavior Cam Fs":dbl)  [unwired: 7 in, 2 out]
        n151 = local read "Analog Data"() -> (w598:bool)
        n152 = local read "stop"() -> (w596:bool)
        n153 = Compound Arithmetic op=OR(w596, w598) -> (w597:bool)
      }
      n154 = while {
        tunnel: [w580] -> w321
        tunnel: [w587] -> w323
        tunnel: w373 -> [w579]
        tunnel: w372 -> [w578]
        tunnel: w371 -> [w577]
        tunnel: w370 -> [w576]
        tunnel: w367 -> [w575]
        tunnel: [w574] -> w322
        tunnel: w365 -> [w574]
        i -> [w588]
        stop <- w582 stop-if-true
        n155 = Tick Count (ms)() -> (millisecond timer value=w592:u32)
        n156 = Greater?(x=w578, y=w588) -> (0:→"MScan Cam":bool)
        n157 = Subtract(x=w592, y=w579) -> (x-y=w593:u32)
        n158 = Divide(x=w593, y=u32 1000) -> (x/y=w586:dbl)
        n159 = call "GrabWebCam_2P.vi"("Session In"=w577, "Image In"=w575, "Trial Time"=w586, "AVI Refnum"=w574, "error in"=w576) -> ("Session Out"=w580:T3, "WebCam Img Out"=→"?":T1, "Buffer Number Out"=w584:u32, "error out"=w587:errorcluster)  [unwired: 7 in]
        n160 = call <vilib>:"Calculate Frames per Second.vi"("Update Interval (ms)"=u32 5000, "Buffer Number"=w584) -> ("Processed Frames/s"=→"MSCan Cam Fs":dbl)  [unwired: 7 in, 2 out]
        n161 = local read "Analog Data"() -> (w583:bool)
        n162 = local read "stop"() -> (w581:bool)
        n163 = Compound Arithmetic op=OR(w581, w583) -> (w582:bool)
      }
      n164 = flat-sequence {
        tunnel: [w562] -> w348
        tunnel: [w561] -> w347
        tunnel: w346 -> [w551]
        tunnel: w345 -> [w560]
        tunnel: w344 -> [w559]
        tunnel: w343 -> [w558]
        tunnel: [w557] -> w342
        tunnel: [w556] -> w341
        tunnel: [w555] -> w340
        tunnel: [w554] -> w339
        tunnel: w338 -> [w553]
        tunnel: w337 -> [w552]
        tunnel: w328 -> [w550]
        tunnel: w327 -> [w549]
        tunnel: w326 -> [w547]
        tunnel: w325 -> [w548]
        tunnel: w324 -> [w546]
        tunnel: w323 -> [w544]
        tunnel: w322 -> [w545]
        tunnel: w321 -> [w543]
        tunnel: [w542] -> w320
        tunnel: [w541] -> w318
        tunnel: w348 -> [w570]
        tunnel: w347 -> [w569]
        tunnel: w342 -> [w568]
        tunnel: w341 -> [w567]
        tunnel: w340 -> [w566]
        tunnel: w339 -> [w565]
        tunnel: w320 -> [w564]
        tunnel: [w564] -> w319
        tunnel: w318 -> [w563]
        tunnel: [w563] -> w317
        frame #0 {
          n165 = call <vilib>:"IMAQdx Close Camera.vi"("error in"=w550, "Session In"=w549) -> ()  [unwired: 9 in, 1 out]
          n166 = call <vilib>:"IMAQdx Close Camera.vi"("error in"=w544, "Session In"=w543) -> ()  [unwired: 9 in, 1 out]
          n167 = call "IMAQ AVI2 Close"("error in (no error)"=w544, "AVI Refnum"=w545) -> ("error out"=w541:errorcluster)  [unwired: 9 in]
          n168 = call <vilib>:"IMAQdx Close Camera.vi"("error in"=w547, "Session In"=w546) -> ()  [unwired: 9 in, 1 out]
          n169 = call "IMAQ AVI2 Close"("error in (no error)"=w547, "AVI Refnum"=w548) -> ("error out"=w542:errorcluster)  [unwired: 9 in]
          n170 = call <vilib>:"DAQmx Stop Task.vi"("task/channels in"=w553, "error in"=w552) -> ("task out"=w555:refnum<k21>, "error out"=w554:errorcluster)  [unwired: 12 in]
          n171 = call <vilib>:"DAQmx Stop Task.vi"("task/channels in"=w551, "error in"=w560) -> ("task out"=w562:refnum<k21>, "error out"=w561:errorcluster)  [unwired: 12 in]
          n172 = call <vilib>:"DAQmx Stop Task.vi"("task/channels in"=w559, "error in"=w558) -> ("task out"=w556:refnum<k21>, "error out"=w557:errorcluster)  [unwired: 12 in]
        }
        frame #1 {
          n173 = call <vilib>:"DAQmx Clear Task.vi"("task in"=w566, "error in"=w565) -> ()  [unwired: 13 in, 1 out]
          n174 = call <vilib>:"DAQmx Clear Task.vi"("task in"=w567, "error in"=w568) -> ()  [unwired: 13 in, 1 out]
          n175 = call <vilib>:"DAQmx Clear Task.vi"("task in"=w570, "error in"=w569) -> ()  [unwired: 13 in, 1 out]
        }
      }
      n176 = Delete From Array(array=w495, length=1, index=0) -> (array with subset deleted=w525:u32[])  [unwired: 1 out]
      n177 = Delete From Array(array=w519, length=1, index=0) -> (array with subset deleted=w526:u32[])  [unwired: 1 out]
      n178 = Close File(refnum=w477, error in=w505) -> (path=w497:path, error out=w498:errorcluster)
      n179 = Move(source path=w364, error in=w319, 10:"Target Path") -> (error out=w414:errorcluster)  [unwired: 2 in, 2 out]
      n180 = Move(source path=w497, error in=w498, 10:"Target Path") -> (error out=w500:errorcluster)  [unwired: 2 in, 2 out]
      n181 = Move(source path=w362, error in=w317, 10:"Target Path") -> (error out=w366:errorcluster)  [unwired: 2 in, 2 out]
      n182 = Build Array(w526, w525) -> (w523:u32[][])
      n183 = Array To Spreadsheet String(delimiter (Tab)=",", array=w526, 3:"%d" ("format string")) -> (spreadsheet string=w515:string)
      n184 = Array To Spreadsheet String(delimiter (Tab)=",", array=w525, 3:"%d" ("format string")) -> (spreadsheet string=w516:string)
      n185 = Transpose 2D Array(2D array=w523) -> (transposed array=w524:u32[][])
      n186 = call <vilib>:"Simple Error Handler.vi"("error in (no error)"=w500) -> ()  [unwired: 1 in, 8 out]
      n187 = call <vilib>:"Simple Error Handler.vi"("error in (no error)"=w414) -> ()  [unwired: 1 in, 8 out]
      n188 = call <vilib>:"Simple Error Handler.vi"("error in (no error)"=w366) -> ()  [unwired: 1 in, 8 out]
      n189 = call <vilib>:"Trim Whitespace.vi"("string"=w515) -> ("trimmed string"=w390:string)  [unwired: 1 in]
      n190 = call <vilib>:"Trim Whitespace.vi"("string"=w516) -> ("trimmed string"=w517:string)  [unwired: 1 in]
      n191 = Number To Decimal String(number=w524) -> ()  [unwired: 1 in, 1 out]
      n192 = Build Array(w390, w517) -> (w518:string[])
      n193 = TDMS Set Properties(5:w518, 7:string[] ["WhiskerCam_DroppedFrameIndex", "WhiskerCam_NumberDropped"] ("channel name(s) in (Untitled)"), 8:w337, 11:w512) -> (0:w513:errorcluster, 3:w514:refnum<k34>)  [unwired: 2 in, 2 out]
      n194 = TDMS Close(8:w513, 11:w514) -> (0:w496:errorcluster, 3:w501:path)
      n195 = Path To String(path=w501) -> (string=w389:string)
      n196 = Concatenate Strings(w389, "_index" ("string")) -> (w502:string)
      n197 = TDMS Defragment(4:w496, 7:w501) -> (0:w504:errorcluster)
      n198 = String To Path(string=w502) -> (path=w503:path)
      n199 = Move(source path=w501, error in=w504, 10:"Target Path") -> (error out=w499:errorcluster)  [unwired: 2 in, 2 out]
      n200 = Move(source path=w503, error in=w504, 10:"Target Path") -> (error out=w388:errorcluster)  [unwired: 2 in, 2 out]
      n201 = call <vilib>:"Simple Error Handler.vi"("error in (no error)"=w388) -> ()  [unwired: 1 in, 8 out]
      n202 = call <vilib>:"Simple Error Handler.vi"("error in (no error)"=w499) -> ()  [unwired: 1 in, 8 out]
    }
    frame #4 {
      "Complete" <- TRUE ("Data Acquisition - Complete")
    }
  }
